vi "ITX to TDMS.vi"(8 "error in (no error)":errorcluster, 11 "file (use dialog)":path=path "C:/") -> (0 "error out":errorcluster)   [LabVIEW 2016]
uses:
  Data/Typedefs/Type--enum.ctl
  Data/Data.lvclass
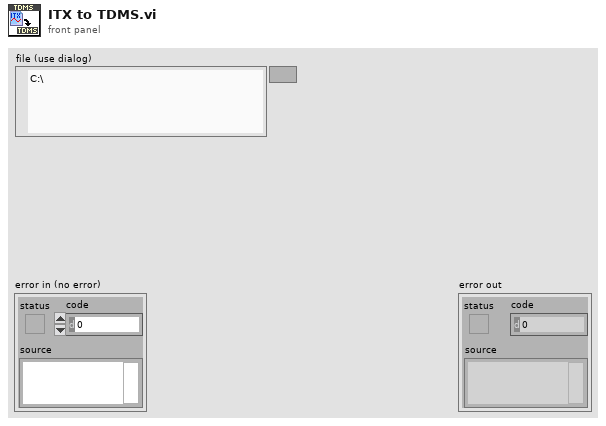
[diagram p1: front panel]
types:
  T1 = typedef "Data.lvclass/Type--enum.ctl" = enum16{"DAT", "ITX", "HDF5", "TDMS", "VI"}
  T2 = typedef "Data.lvclass/Dictionary--cluster.ctl" = cluster{"key":string, "value":variant}
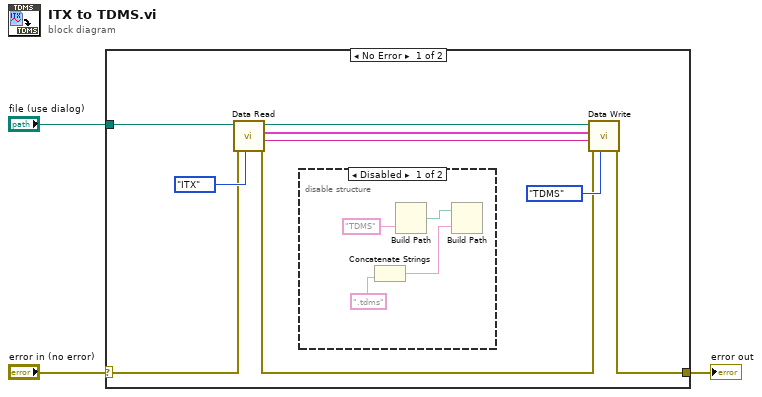
[diagram p0: block diagram]
diagram:
  n1 = case shown="No Error" "error in (no error)" {
    selector: "error in (no error)" -> [w9 w19]
    tunnel: [w7 w19] -> w2
    tunnel: "file (use dialog)" -> [w12 _]
    frame No Error {
      n2 = call "Data Read.vi"("File Type"=Type--enum."ITX", "error in (no error)"=w9, "path"=w12) -> ("error out"=w4:errorcluster, "Notes"=w5:string, "Data (Dictionary)"=w6:T2[], "path out"=w8:path)  [unwired: 5 in]
      n3 = disable-structure shown="Disabled" {
        frame Disabled {
          n4 = Concatenate Strings(".tdms" ("string")) -> (w17:string, w18:string)
          n5 = Build Path(name or relative path="TDMS" ("string")) -> (base path=w13:path, appended path=w14:path)
          n6 = Build Path(base path=w14, name or relative path=w17) -> ()  [unwired: 1 out]
        }
        frame Enabled {
        }
      }
      n7 = call "Data Write.vi"("File Type"=Type--enum."TDMS", "error in (no error)"=w4, "Notes"=w5, "Data (Dictionary)"=w6, "path"=w8) -> ("error out"=w7:errorcluster)  [unwired: 5 in, 1 out]
    }
    frame Error {
    }
  }
  "error out" <- w2
